vi "templates decode import content.vi"(8 "error in (no error)":errorcluster, 10 "Valid Content-Type: (\"text/xml\")":string="text/xml", 11 "Multi-Part Content (\"\")":string) -> (0 "error out":errorcluster, 3 "Content":string)   [LabVIEW 2011]
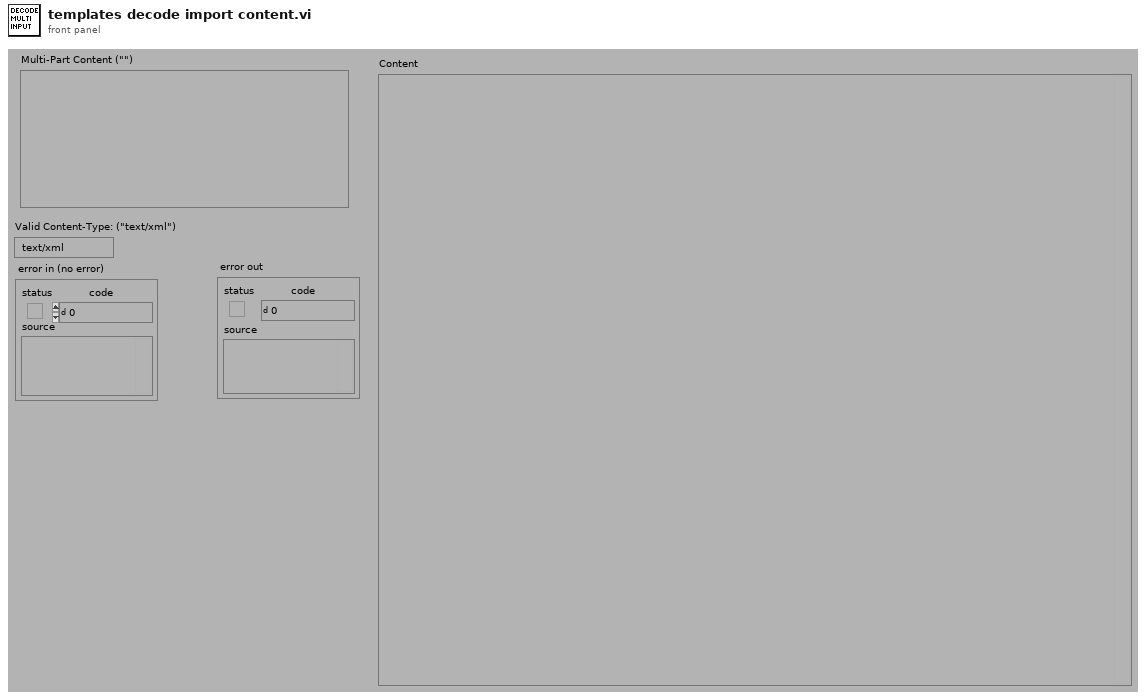
[diagram p1: front panel]
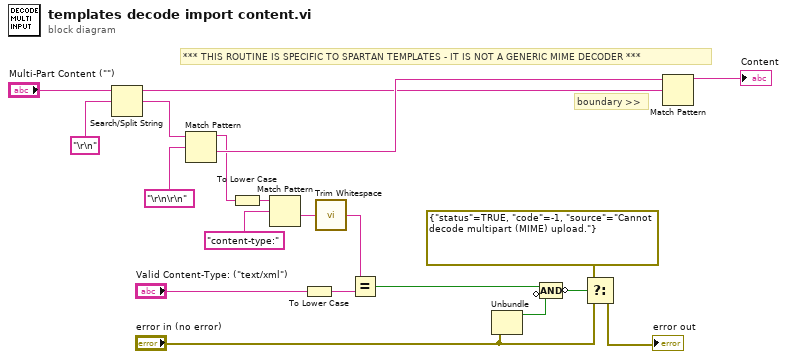
[diagram p0: block diagram]
diagram:
  # "*** THIS ROUTINE IS SPECIFIC TO SPARTAN TEMPLATES - IT IS NOT A GENERIC MIME DECODER ***"
  # "boundary >>"
  n1 = Search/Split String(string="Multi-Part Content (\"\")", search string/char (-)="\r\n" ("regular expression")) -> (substring before match=w1:string, match + rest of string=w2:string)  [unwired: 1 in, 1 out]
  n2 = Match Pattern(string=w2, regular expression="\r\n\r\n") -> (before substring=w9:string, after substring=w19:string)  [unwired: 3 out]
  n3 = To Lower Case(string=w9) -> (all lower case string=w10:string)
  n4 = Match Pattern(string=w10, regular expression="content-type:") -> (after substring=w7:string)  [unwired: 4 out]
  n5 = To Lower Case(string="Valid Content-Type: (\"text/xml\")") -> (all lower case string=w12:string)
  n6 = call <vilib>:"Trim Whitespace.vi"("string"=w7) -> ("trimmed string"=w6:string)  [unwired: 1 in]
  n7 = Equal?(x=w6, y=w12) -> (x = y?=w5:bool)
  n8 = Unbundle("error in (no error)") -> ("status"=w16:bool)  [unwired: 2 out]
  n9 = Compound Arithmetic op=AND(w5, invert w16) -> (invert w17:bool)
  n10 = Select(t=errorcluster {"status"=TRUE, "code"=-1, "source"="Cannot decode multipart (MIME) upload."}, s=w17, f="error in (no error)") -> (s? t:f=→"error out":errorcluster)
  n11 = Match Pattern(string=w19, regular expression=w1) -> (before substring=→"Content":string)  [unwired: 4 out]
